vi "shutdown.vi"(8 "error in (no error)":errorcluster, 11 "VISA resource name":refnum<visa-resource-name>="COM9") -> (0 "error out":errorcluster, 2 "write buffer":string="SD\r\n", 3 "VISA resource name out":refnum<visa-resource-name>="COM9")   [LabVIEW 2017, in "radiant.lvlib"]
doc: "<B>Laser Goto with FCU</B> VI tunes laser to the position <B>Wavenumber (1/cm)</B>. FCU1 is adjusted accordingly."
uses:
  <vilib>/Instr/_visa.llb/VISA Configure Serial Port (Instr).vi
  radiant.lvlib
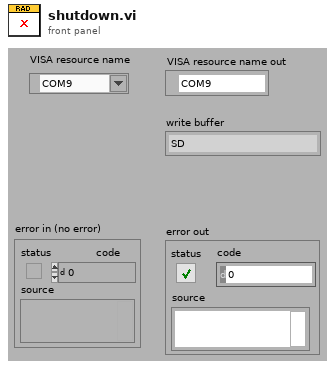
[diagram p1: front panel]
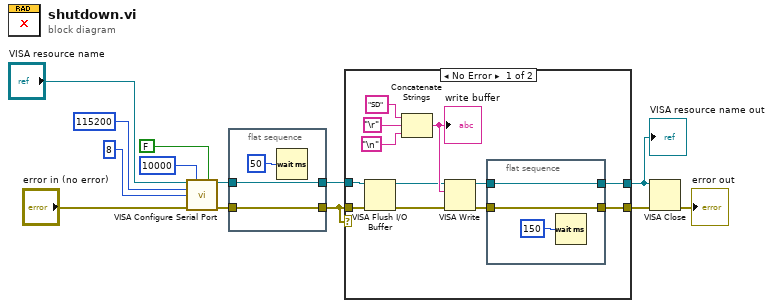
[diagram p0: block diagram]
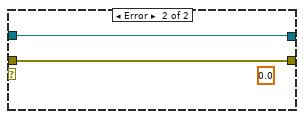
[diagram p2: hidden frame]
diagram:
  n1 = call-poly "VISA Configure Serial Port"("VISA resource name"="VISA resource name", "timeout (10sec)"=u32 10000, "Enable Termination\nChar (T)"=FALSE ("Enable Termination\nChar (T)"), "baud rate (9600)"=u32 115200, "data bits (8)"=u16 8, "error in (no error)"="error in (no error)") -> ("VISA resource name out"=w6:refnum<visa-resource-name>, "error out"=w4:errorcluster)  [unwired: 8 in]
  n2 = flat-sequence {
    tunnel: w6 -> [w16]
    tunnel: [w16] -> w5
    tunnel: w4 -> [w15]
    tunnel: [w15] -> w3
    frame #0 {
      n3 = Wait (ms)(milliseconds to wait=u32 50) -> ()  [unwired: 1 out]
    }
  }
  n4 = case shown="No Error" w3 {
    tunnel: w3 -> [w25 w33]
    tunnel: w5 -> [w24 w32]
    tunnel: [w19 w33] -> w1
    tunnel: [w18 w32] -> w2
    frame No Error {
      n5 = VISA Flush I/O Buffer(VISA resource name=w24, error in (no error)=w25) -> (VISA resource name out=w23:refnum<visa-resource-name>, error out=w22:errorcluster)  [unwired: 1 in]
      n6 = Concatenate Strings("SD" ("write"), "\r", "\n") -> (w26:string)
      "write buffer" <- w26
      n7 = VISA Write(VISA resource name=w23, write buffer=w26, error in (no error)=w22) -> (VISA resource name out=w21:refnum<visa-resource-name>, error out=w20:errorcluster)  [unwired: 1 out]
      n8 = flat-sequence {
        tunnel: w21 -> [w31]
        tunnel: [w31] -> w18
        tunnel: w20 -> [w30]
        tunnel: [w30] -> w19
        frame #0 {
          n9 = Wait (ms)(milliseconds to wait=u32 150) -> ()  [unwired: 1 out]
        }
      }
    }
    frame Error {
      (unwired) 0.0
    }
  }
  "VISA resource name out" <- w2
  n10 = VISA Close(VISA resource name=w2, error in (no error)=w1) -> (error out=→"error out":errorcluster)
